vi "Heat Flow Front Panel.vi"() -> ()   [LabVIEW 2019, in "Results.lvlib" / "Heat Flow Results.lvclass"]
uses:
  Heat Flow Results.lvclass
  Heat Flow Results.lvclass/Heat Flow Results.ctl
  Test Stands/Heat Flow/Heat Flow Test Stand.lvclass
panel:
  in  "Ugs Hot":dbl min=0.0 max=10.0 step=0.1
  out "Gas Humidity":dbl caption="Air Humid" format="%#.4f"
  out "Adjusted":bool
  in  "Heater Temp SP":dbl min=0.0 max=372.0 step=1.0
  in  "auto Flow":bool
  in  "Ugs Cold":dbl min=0.0 max=10.0 step=0.1
  in  "Heater Power SP":dbl min=0.0 max=300.0 step=1.0
  in  "auto pwr":bool
  out "Gas Flow":dbl format="%#.3f"
  out "Gas Speed":dbl caption="Gas Linear Speed" format="%#.4f"
  out "U Load":dbl format="%#.2f"
  out "P Heater":dbl format="%#.2f"
  out "I Heater":dbl format="%#.2f"
  out "I Load":dbl format="%#.2f"
  out "P TEG":dbl format="%#.2f"
  out "Data":dbl(graph) caption="Pressure drops"
  # "Heat Flow Test Stand"
  # "Automatic"
  # "Manual"
  # "Falownik"
  # "FTCU 100"
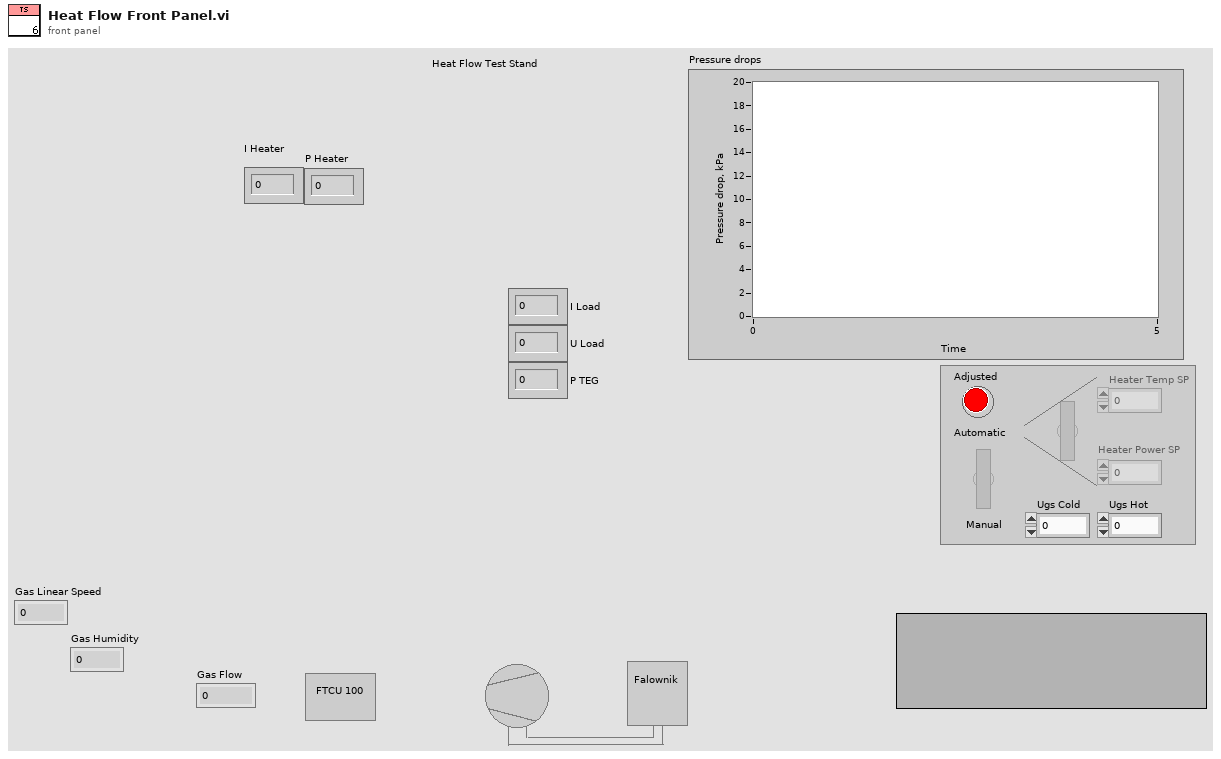
[diagram p1: front panel]
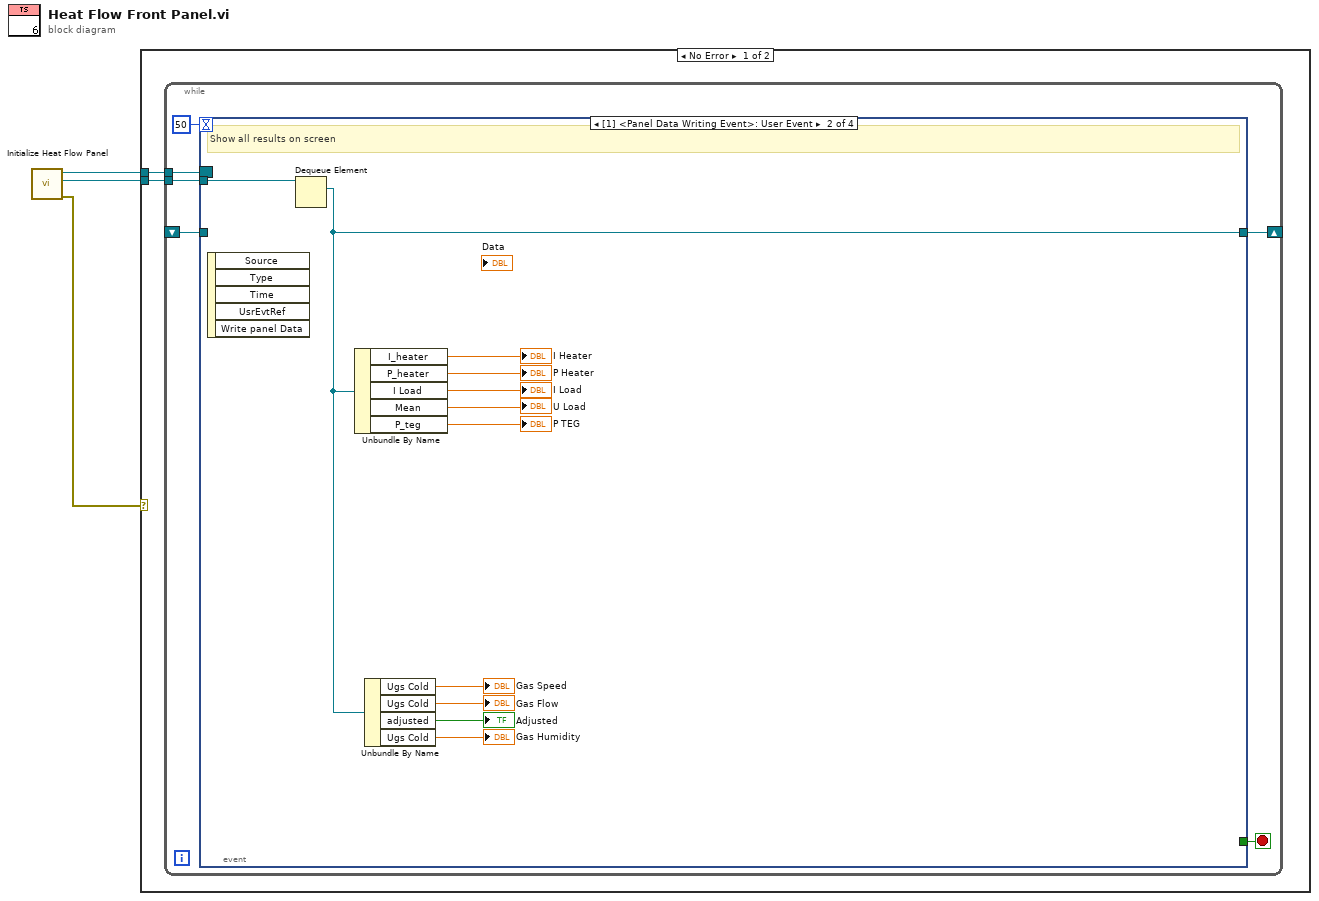
[diagram p0: block diagram]
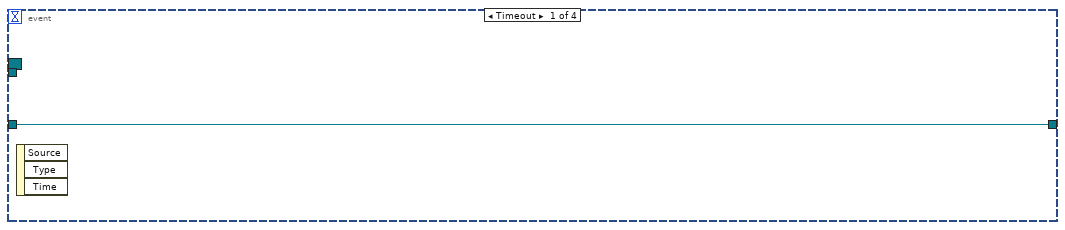
[diagram p2: hidden frame]
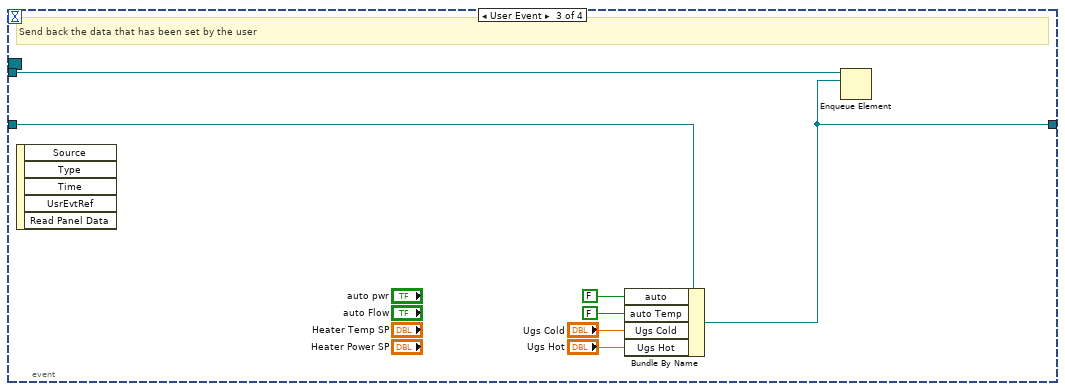
[diagram p3: hidden frame]
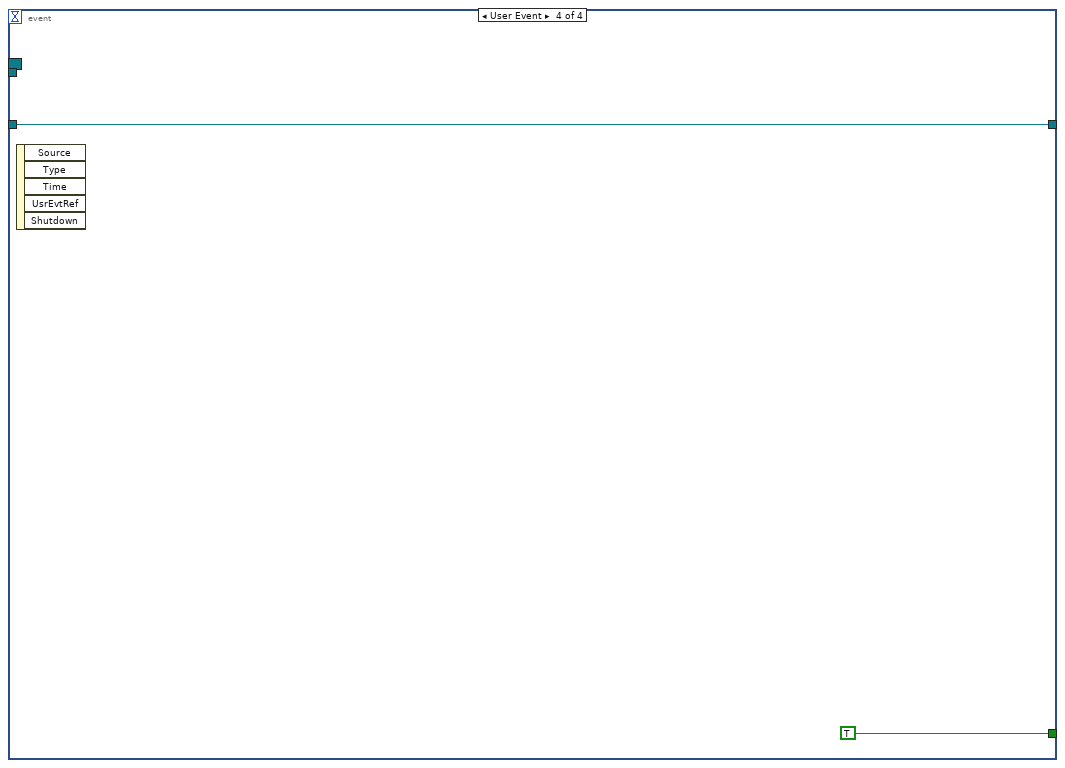
[diagram p4: hidden frame]
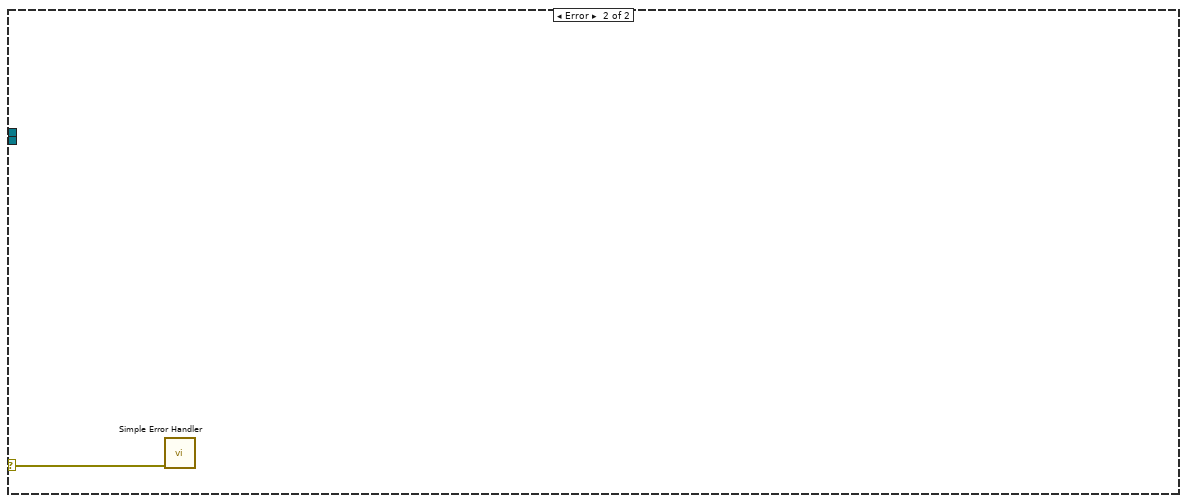
[diagram p5: hidden frame]
diagram:
  n1 = call "Initialize Heat Flow Panel.vi"() -> ("error out"=w3:errorcluster, "Heat Flow Results queue out"=w1:refnum<queue>, "Event Registration Refnum"=w2:refnum<event-registration>)  [unwired: 9 in]
  n2 = case shown="No Error" w3 {
    selector: w3 -> [_ w33]
    tunnel: w2 -> [w5 _]
    tunnel: w1 -> [w4 _]
    frame No Error {
      n3 = while {
        tunnel: w5 -> [w10]
        tunnel: w4 -> [w9]
        shift-right: [w7] -> _
        shift-left: _ -> [w6]
        stop <- w11 stop-if-true
        n4 = event shown="[1] <Panel Data Writing Event>: User Event" {
          selector: w10 -> [_ _ _ _]
          dyn-events: _ -> [_ _ _ _]
          timeout: 50 -> [_ _ _ _]
          tunnel: [_ _ _ TRUE] -> w11
          tunnel: w9 -> [_ w23 w30 _]
          tunnel: [w12 w22 w28 w31] -> w7
          tunnel: w6 -> [w12 _ w29 w31]
          event Timeout {
            n5 = event-data() -> ()  [unwired: 1 in, 3 out]
          }
          event User Event {
            # "Show all results on screen"
            n6 = event-data() -> ()  [unwired: 1 in, 5 out]
            n7 = Dequeue Element(queue=w23) -> (element=w22:refnum<class "Heat Flow Results.lvclass">)  [unwired: 2 in, 3 out]
            n8 = Unbundle By Name(w22) -> ("I_heater"=→"I Heater":dbl, "P_heater"=→"P Heater":dbl, "I Load"=→"I Load":dbl, "Mean"=→"U Load":dbl, "P_teg"=→"P TEG":dbl)
            n9 = Unbundle By Name(w22) -> ("Ugs Cold"=→"Gas Speed":dbl, "Ugs Cold"=→"Gas Flow":dbl, "adjusted"=→"Adjusted":bool, "Ugs Cold"=→"Gas Humidity":dbl)
          }
          event User Event {
            # "Send back the data that has been set by the user"
            n10 = event-data() -> ()  [unwired: 1 in, 5 out]
            n11 = Bundle By Name(cluster=w29, "auto"=FALSE, "auto Temp"=FALSE, "Ugs Cold"="Ugs Cold", "Ugs Hot"="Ugs Hot") -> (w28:refnum<class "Heat Flow Results.lvclass">)
            n12 = Enqueue Element(queue=w30, element=w28) -> ()  [unwired: 2 in, 3 out]
          }
          event User Event {
            n13 = event-data() -> ()  [unwired: 1 in, 5 out]
          }
        }
      }
    }
    frame Error {
      n14 = call <vilib>:"Simple Error Handler.vi"("error in (no error)"=w33) -> ()  [unwired: 4 in, 5 out]
    }
  }
